vi "Set Test information.vi"(4 "Test Information In":T1={"Scan barcode"=FALSE, "Length"=0, "Test Station Code"="", "Environment"="", "Inspector"="", "Customer Name"="", "Order Number"="", "Fail Rate Max"=0.0, "Repeat"=10}) -> (1 "Test Information":T1={"Scan barcode"=FALSE, "Length"=0, "Test Station Code"="", "Environment"="", "Inspector"="", "Customer Name"="", "Order Number"="", "Fail Rate Max"=0.0, "Repeat"=10})   [LabVIEW 2018]
uses:
  <vilib>/Utility/config.llb/Write Key (String).vi
  <vilib>/Utility/config.llb/NI_LVConfig.lvlib
panel:
  in  "保存路径":bool
  in  "customname 2":string caption="夹具编号"
  out "元素 4":bool
  out "元素 3":bool
  out "元素 2":bool
  out "元素":bool
  in  "XML":bool
  in  "TXT":bool
  in  "CSV":bool
  in  "MES":bool
  out "数组":string[](array[string])
  out "添加的路径":path
  out "添加的数组":string[](array[string])
  out "布尔":bool
  in  "Bar":bool
  out "exit":bool
  in  "重测":i32=10 caption="Max"
  in  "count":string caption="检 验 员"
  in  "SCAN":bool
  in  "长度":u8=8 min=1
  in  "不超过":dbl=10.0 caption="Max" format="%#.2f"
  in  "Cancel":bool
  in  "OK":bool
  in  "envirment":string caption="测试环境"
  in  "order":string caption="工    令"
  in  "customname":string caption="测试计数"
  in  "是否扫条形码":bool
  # "SetTestInformaton"
  # "不良率报警设置"
  # "信息设置"
  # "字符"
  # "%"
  # "提示：勾选了扫描条码，但其长度设置为0表示不校验输入条码。"
  # "数据保存位置"
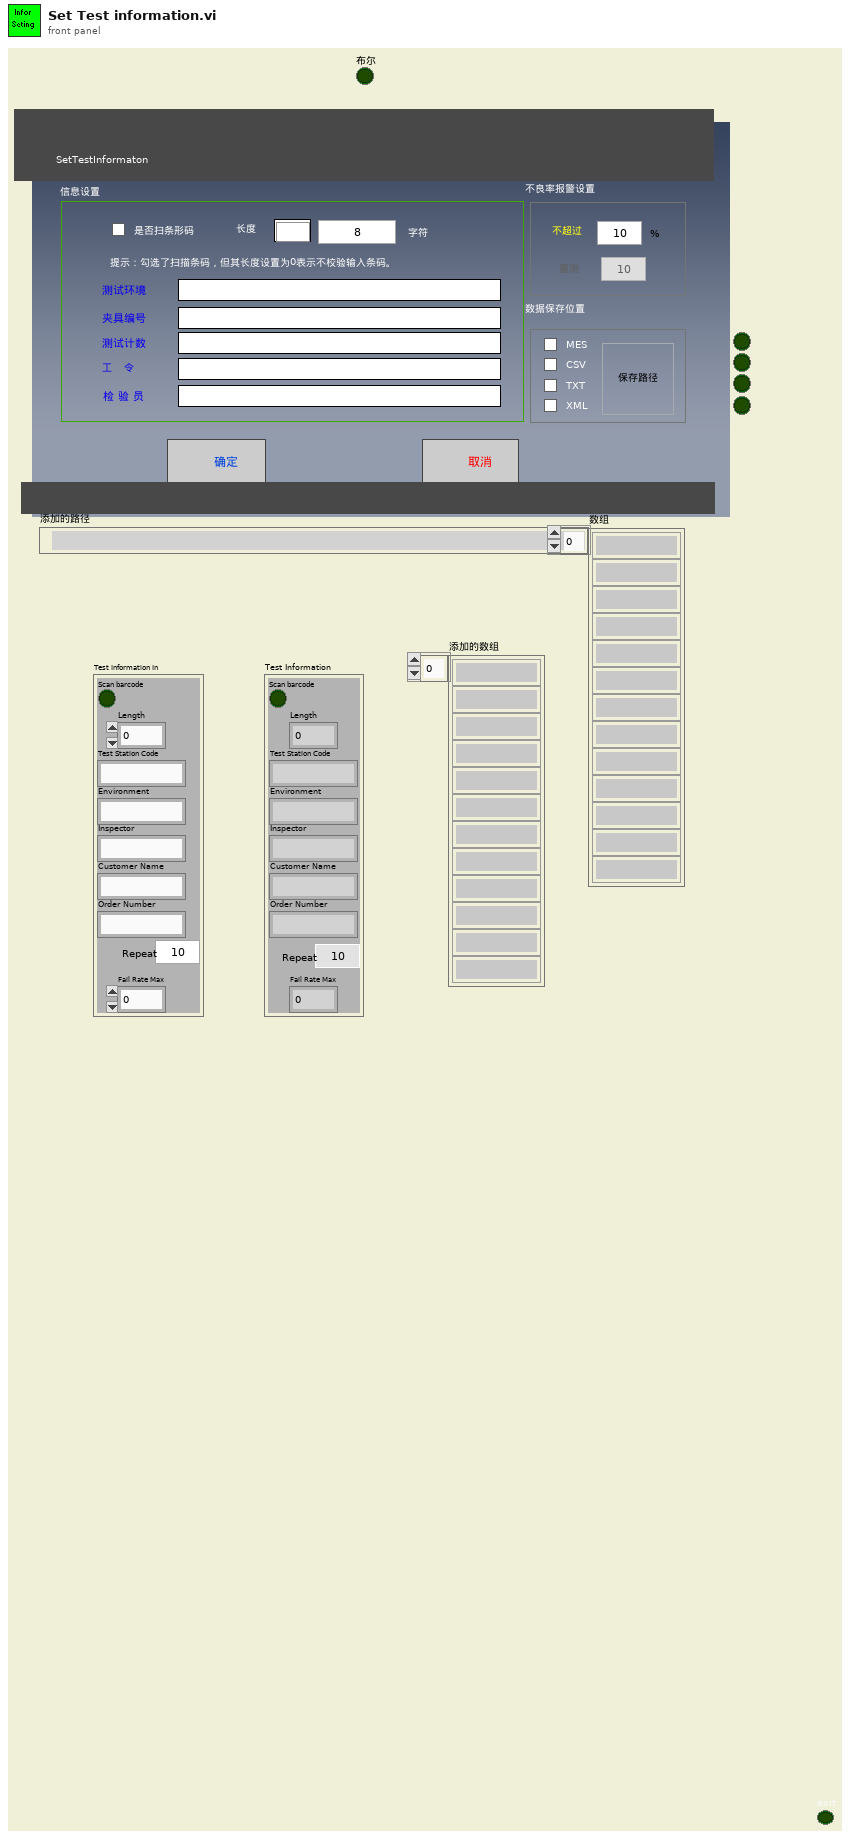
[diagram p1: front panel]
types:
  T1 = cluster{"Scan barcode":bool, "Length":u8, "Test Station Code":string, "Environment":string, "Inspector":string, "Customer Name":string, "Order Number":string, "Fail Rate Max":dbl, "Repeat":i32}
  T2 = typedef "NI_LVConfig.lvlib/Config Data RefNum.ctl" = refnum<k1>
  T3 = cluster{"Scan barcode":bool, "Length":u8, "Test Station Code":string, "Environment":string, "Inspector":string, "Customer Name":string, "Order Number":string, "Fail Rate Max":dbl, "repeat":i32}
  T4 = typedef "Window Refnum.ctl" = refnum<k1>
  T5 = typedef "Window Rectangle.ctl" = cluster{"left":i16, "top":i16, "right":i16, "bottom":i16}
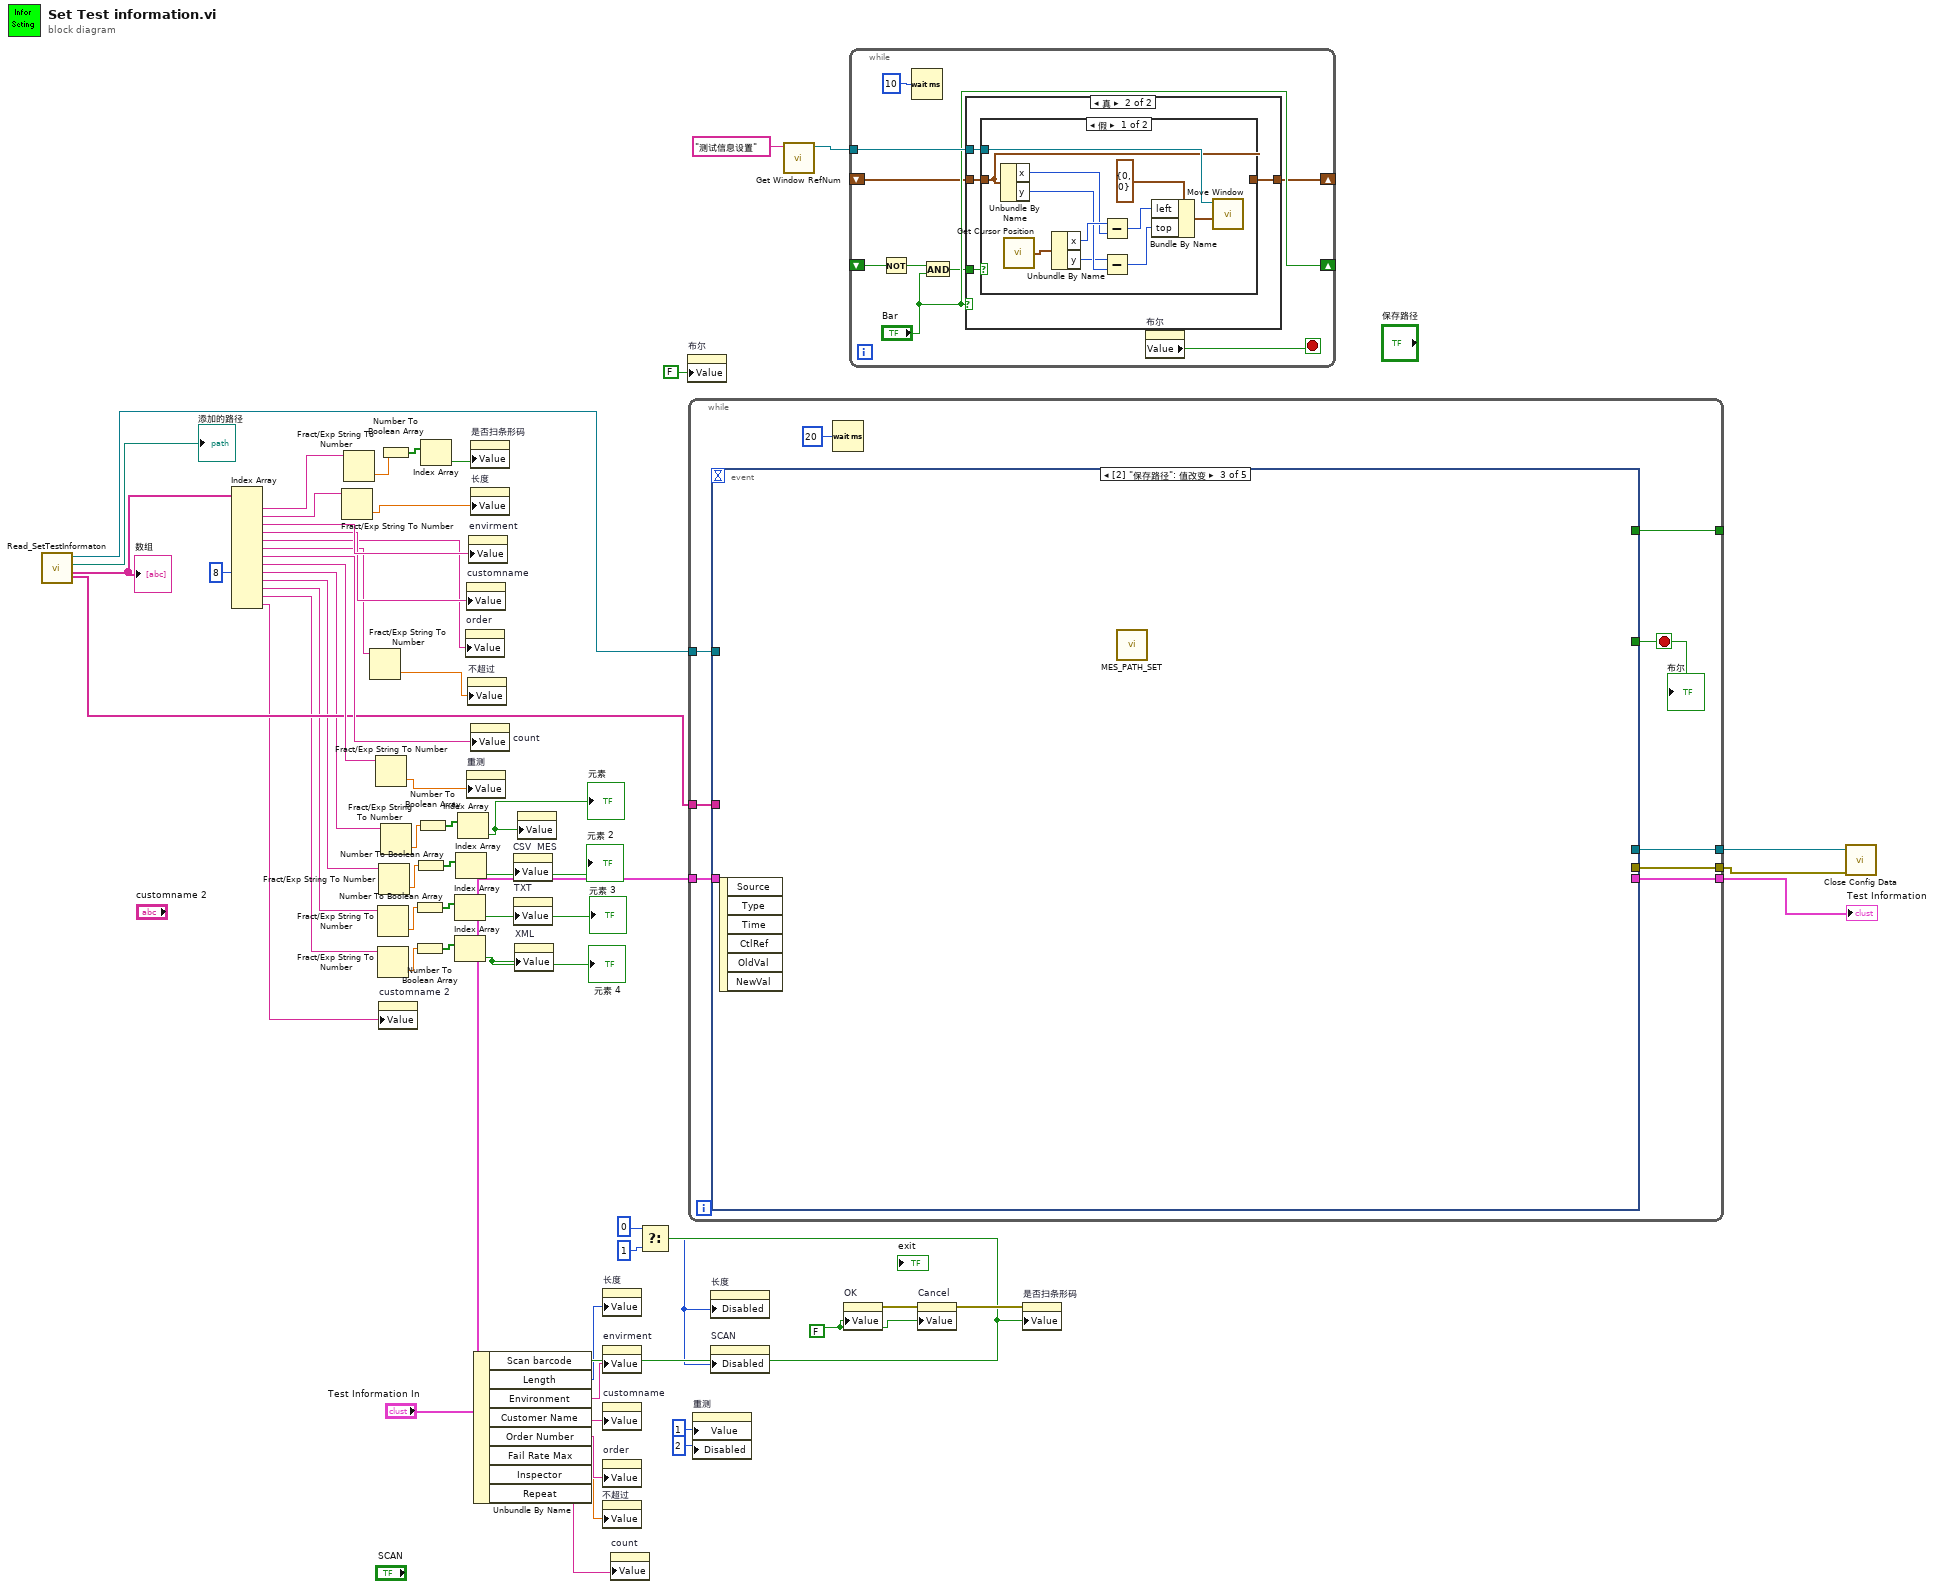
[diagram p0: block diagram]
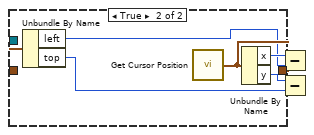
[diagram p3: hidden frame]
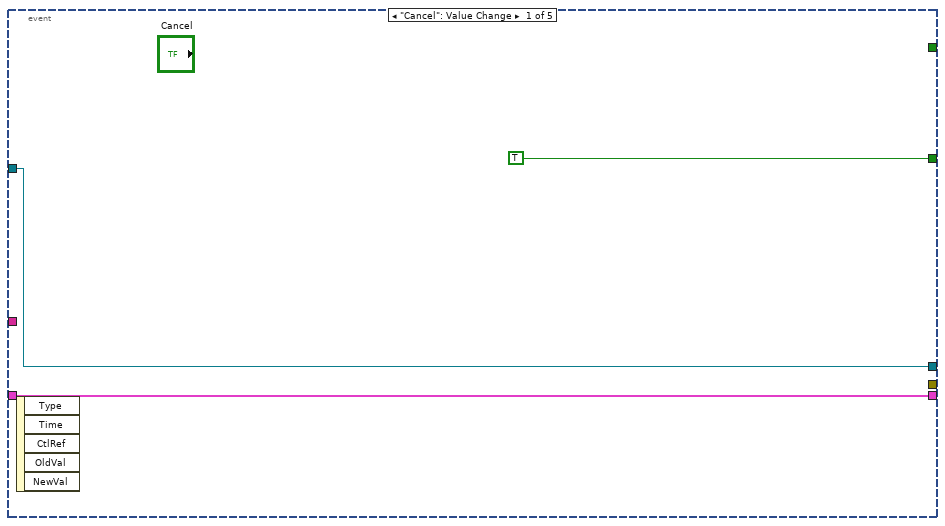
[diagram p4: hidden frame]
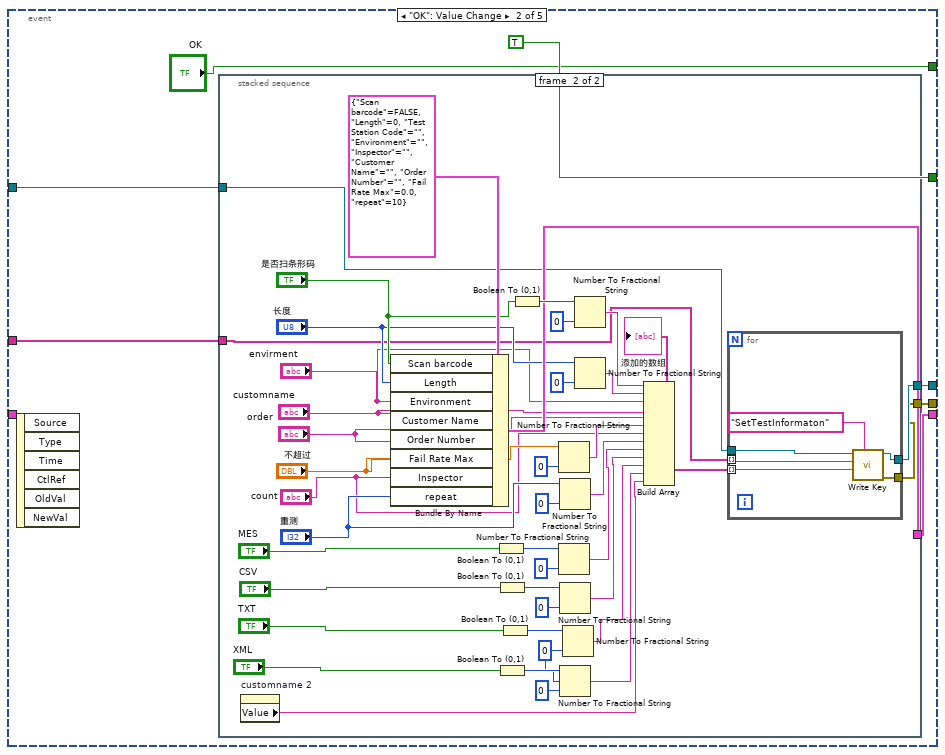
[diagram p5: hidden frame]
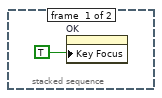
[diagram p6: hidden frame]
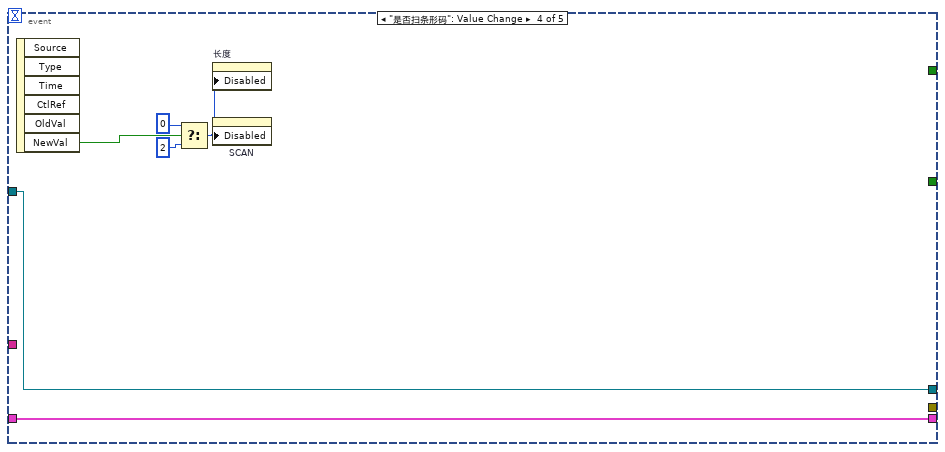
[diagram p7: hidden frame]
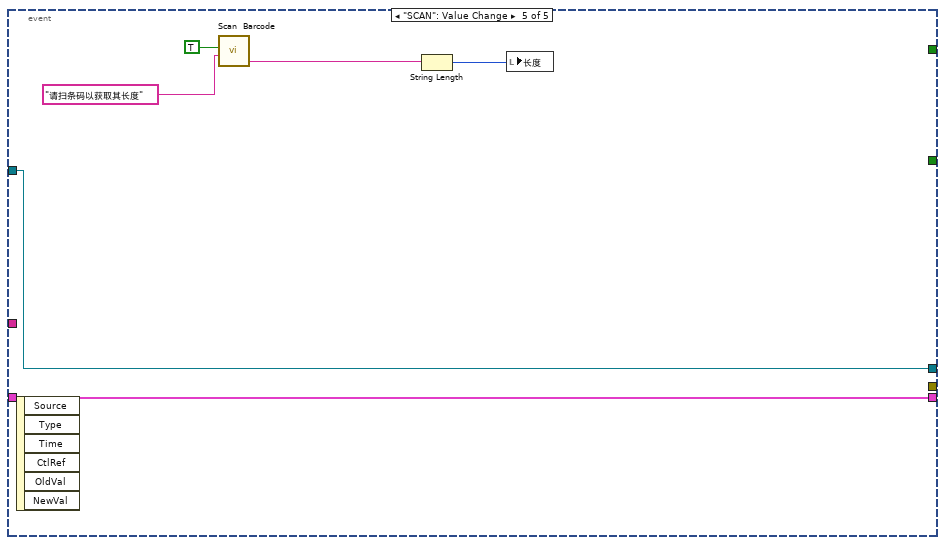
[diagram p8: hidden frame]
diagram:
  w57 = FALSE
  n1 = call "Read_SetTestInformaton.vi"() -> ("数组 2"=w36:string[], "appended path"=→"添加的路径":path, "引用句柄输出"=w37:T2, "数组"=w21:string[])  [unwired: 7 in, 1 out]
  "数组" <- w36
  n2 = Index Array(array=w36, index #9=8 ("索引")) -> (element #1=w35:string, element #2=w31:string, element #3=w29:string, element #4=w28:string, element #5=w27:string, element #6=w25:string, element #7=w24:string, element #8=w22:string, element #9=w14:string, element #10=w13:string, element #11=w12:string, element #12=w11:string, element #13=w1:string)  [unwired: 12 in]
  n3 = Fract/Exp String To Number(string=w31) -> (number=w30:dbl)  [unwired: 3 in, 1 out]
  n4 = Fract/Exp String To Number(string=w35) -> (number=w34:dbl)  [unwired: 3 in, 1 out]
  n5 = Fract/Exp String To Number(string=w25) -> (number=w26:dbl)  [unwired: 3 in, 1 out]
  n6 = Fract/Exp String To Number(string=w22) -> (number=w23:dbl)  [unwired: 3 in, 1 out]
  n7 = Fract/Exp String To Number(string=w12) -> (number=w3:dbl)  [unwired: 3 in, 1 out]
  n8 = Fract/Exp String To Number(string=w11) -> (number=w2:dbl)  [unwired: 3 in, 1 out]
  n9 = Fract/Exp String To Number(string=w13) -> (number=w4:dbl)  [unwired: 3 in, 1 out]
  n10 = property on="customname 2" class="Str"("Value"=w1) -> ()  [unwired: 2 in, 2 out]
  n11 = Number To Boolean Array(number=w34) -> (Boolean array=w33:bool[])
  n12 = Fract/Exp String To Number(string=w14) -> (number=w5:dbl)  [unwired: 3 in, 1 out]
  n13 = Number To Boolean Array(number=w3) -> (Boolean array=w16:bool[])
  n14 = Number To Boolean Array(number=w2) -> (Boolean array=w15:bool[])
  n15 = Number To Boolean Array(number=w4) -> (Boolean array=w17:bool[])
  n16 = Number To Boolean Array(number=w5) -> (Boolean array=w18:bool[])
  n17 = Index Array(array=w33) -> (element=w32:bool)  [unwired: 1 in]
  n18 = Index Array(array=w16) -> (element=w9:bool)  [unwired: 1 in]
  "元素 3" <- w9
  n19 = Index Array(array=w15) -> (element=w10:bool)  [unwired: 1 in]
  "元素 4" <- w10
  n20 = Index Array(array=w17) -> (element=w8:bool)  [unwired: 1 in]
  "元素 2" <- w8
  n21 = Index Array(array=w18) -> (element=w7:bool)  [unwired: 1 in]
  "元素" <- w7
  n22 = property on="order" class="Str"("Value"=w27) -> ()  [unwired: 2 in, 2 out]
  n23 = property on="customname" class="Str"("Value"=w28) -> ()  [unwired: 2 in, 2 out]
  n24 = property on="重测" class="DigNum (严格)"("Value"=w23) -> ()  [unwired: 2 in, 2 out]
  n25 = property on="不超过" class="DigNum (严格)"("Value"=w26) -> ()  [unwired: 2 in, 2 out]
  n26 = property on="envirment" class="Str"("Value"=w29) -> ()  [unwired: 2 in, 2 out]
  n27 = property on="是否扫条形码" class="Bool (严格)"("Value"=w32) -> ()  [unwired: 2 in, 2 out]
  n28 = property on="长度" class="DigNum (严格)"("Value"=w30) -> ()  [unwired: 2 in, 2 out]
  n29 = property on="count" class="Str"("Value"=w24) -> ()  [unwired: 2 in, 2 out]
  n30 = Unbundle By Name("Test Information In") -> ("Scan barcode"=w51:bool, "Length"=w47:u8, "Environment"=w56:string, "Customer Name"=w55:string, "Order Number"=w54:string, "Fail Rate Max"=w46:dbl, "Inspector"=w45:string)  [unwired: 1 out]
  n31 = property on="CSV" class="Bool (严格)"("Value"=w8) -> ()  [unwired: 2 in, 2 out]
  n32 = property on="TXT" class="Bool (严格)"("Value"=w9) -> ()  [unwired: 2 in, 2 out]
  n33 = property on="XML" class="Bool (严格)"("Value"=w10) -> ()  [unwired: 2 in, 2 out]
  n34 = property on="MES" class="Bool (严格)"("Value"=w7) -> ()  [unwired: 2 in, 2 out]
  n35 = property on="长度" class="DigNum (严格)"("Value"=w47) -> ()  [unwired: 2 in, 2 out]
  n36 = property on="envirment" class="Str"("Value"=w56) -> ()  [unwired: 2 in, 2 out]
  n37 = property on="customname" class="Str"("Value"=w55) -> ()  [unwired: 2 in, 2 out]
  n38 = property on="order" class="Str"("Value"=w54) -> ()  [unwired: 2 in, 2 out]
  n39 = property on="不超过" class="DigNum (严格)"("Value"=w46) -> ()  [unwired: 2 in, 2 out]
  n40 = property on="count" class="Str"("Value"=w45) -> ()  [unwired: 2 in, 2 out]
  n41 = Select(t=u8 0 ("禁用"), s=w51, f=u8 1 ("禁用")) -> (s? t:f=w48:u8)
  n42 = property on="布尔" class="Bool (严格)"("Value"=FALSE ("布尔")) -> ()  [unwired: 2 in, 2 out]
  n43 = while {
    tunnel: [w62] -> w39
    tunnel: "Test Information In" -> [w65]
    tunnel: [w64] -> _
    tunnel: w37 -> [w59]
    tunnel: w21 -> [w63]
    tunnel: [w61] -> w20
    tunnel: [w60] -> w19
    stop <- w66 stop-if-true
    n44 = event shown="[2] \"保存路径\": 值改变" {
      selector: _ -> [_ _ _ _ _]
      dyn-events: _ -> [_ _ _ _ _]
      timeout: _ -> [_ _ _ _ _]
      tunnel: [TRUE TRUE _ _ _] -> w66
      tunnel: [w69 w71 _ w127 w135] -> w62
      tunnel: w65 -> [w69 _ _ w127 w135]
      tunnel: [_ "OK" _ _ _] -> w64
      tunnel: w63 -> [_ w75 _ _ _]
      tunnel: [w68 w74 _ w126 w132] -> w61
      tunnel: [_ w73 _ _ _] -> w60
      tunnel: w59 -> [w68 w72 _ w126 w132]
      event "Cancel": Value Change {
        n45 = event-data() -> ()  [unwired: 6 out]
      }
      event "OK": Value Change {
        n46 = event-data() -> ()  [unwired: 7 out]
        n47 = stacked-sequence {
          tunnel: w75 -> [_ w100]
          tunnel: [_ w109] -> w74
          tunnel: [_ w108] -> w73
          tunnel: w72 -> [_ w101]
          tunnel: [_ w107] -> w71
          frame #0 {
            n48 = property on="OK" class="Bool (严格)"("Key Focus"=TRUE) -> ()  [unwired: 2 in, 2 out]
          }
          frame #1 {
            w88 = i16 0 ("精度(6)")
            n49 = property on="customname 2" class="Str"() -> ("Value"=w79:string)  [unwired: 2 in, 2 out]
            n50 = Bundle By Name(cluster=T3 {"Scan barcode"=FALSE, "Length"=0, "Test Station Code"="", "Environment"="", "Inspector"="", "Customer Name"="", "Order Number"="", "Fail Rate Max"=0.0, "repeat"=10} ("Test Information In 2"), "Scan barcode"="是否扫条形码", "Length"="长度", "Environment"="envirment", "Customer Name"="customname", "Order Number"="order", "Fail Rate Max"="不超过", "Inspector"="count", "repeat"="重测") -> (w107:T3)
            n51 = Boolean To (0,1)(Boolean="MES") -> (0, 1=w94:i16)
            n52 = Boolean To (0,1)(Boolean="CSV") -> (0, 1=w93:i16)
            n53 = Boolean To (0,1)(Boolean="XML") -> (0, 1=w90:i16)
            n54 = Boolean To (0,1)(Boolean="TXT") -> (0, 1=w91:i16)
            n55 = Boolean To (0,1)(Boolean="是否扫条形码") -> (0, 1=w114:i16)
            n56 = Number To Fractional String(number="不超过", precision (6)=i16 0 ("精度(6)")) -> (F-format string=w97:string)  [unwired: 2 in]
            n57 = Number To Fractional String(number=w94, precision (6)=i16 0 ("精度(6)")) -> (F-format string=w87:string)  [unwired: 2 in]
            n58 = Number To Fractional String(number="重测", precision (6)=i16 0 ("精度(6)")) -> (F-format string=w117:string)  [unwired: 2 in]
            n59 = Number To Fractional String(number=w93, precision (6)=i16 0 ("精度(6)")) -> (F-format string=w86:string)  [unwired: 2 in]
            n60 = Number To Fractional String(number=w90, width (-)=w88, precision (6)=i16 0 ("精度(6)")) -> (F-format string=w84:string)  [unwired: 1 in]
            n61 = Number To Fractional String(number=w91, precision (6)=w88) -> (F-format string=w85:string)  [unwired: 2 in]
            n62 = Number To Fractional String(number=w114, precision (6)=i16 0 ("精度(6)")) -> (F-format string=w115:string)  [unwired: 2 in]
            n63 = Number To Fractional String(number="长度", precision (6)=i16 0 ("精度(6)")) -> (F-format string=w116:string)  [unwired: 2 in]
            n64 = Build Array(w115, w116, "envirment", "customname", "order", w97, "count", w117, w87, w86, w85, w84, w79) -> (w118:string[])
            "添加的数组" <- w118
            n65 = for {
              tunnel: w100 -> [w124] mode=indexing
              tunnel: w118 -> [w125] mode=indexing
              tunnel: [w122] -> w109
              tunnel: [w121] -> w108
              tunnel: w101 -> [w120]
              n66 = call-poly <vilib>:"Write Key.vi"("section"="SetTestInformaton", "value"=w125, "key"=w124, "refnum"=w120) -> ("error out"=w121:errorcluster, "refnum out"=w122:T2)  [unwired: 5 in, 1 out]
            }
          }
        }
      }
      event "保存路径": Value Change {
        n67 = event-data() -> ()  [unwired: 7 out]
        n68 = call "MES_PATH_SET.vi"() -> ()  [unwired: 12 in]
      }
      event "是否扫条形码": Value Change {
        n69 = event-data() -> ("NewVal"=w131:bool)  [unwired: 6 out]
        n70 = Select(t=u8 0 ("禁用"), s=w131, f=u8 2 ("禁用")) -> (s? t:f=w128:u8)
        n71 = property on="长度" class="DigNum (严格)"("Disabled"=w128) -> ()  [unwired: 2 in, 2 out]
        n72 = property on="SCAN" class="Bool"("Disabled"=w128) -> ()  [unwired: 2 in, 2 out]
      }
      event "SCAN": Value Change {
        n73 = event-data() -> ()  [unwired: 7 out]
        n74 = call "Scan  Barcode.vi"("前面板窗口:标题"="请扫条码以获取其长度", "no check?"=TRUE ("检查否")) -> ("SN"=w137:string)  [unwired: 2 in, 2 out]
        n75 = String Length(string=w137) -> (length=w136:i32)
        n76 = local write "长度"(w136) -> ()
      }
    }
    "布尔" <- w66
    n77 = Wait (ms)(milliseconds to wait=u32 20) -> ()  [unwired: 1 out]
  }
  "Test Information" <- w39
  n78 = property on="重测" class="DigNum (严格)"("Value"=1 ("重测"), "Disabled"=u8 2 ("禁用")) -> ()  [unwired: 2 in, 2 out]
  n79 = property on="长度" class="DigNum (严格)"("Disabled"=w48) -> ()  [unwired: 2 in, 2 out]
  n80 = property on="SCAN" class="Bool"("Disabled"=w48) -> ()  [unwired: 2 in, 2 out]
  n81 = call "Get Window RefNum.vi"("window name (\"\")"="测试信息设置" ("window name (\"\")")) -> ("window refnum (NaWR)"=w41:T4)  [unwired: 1 in, 7 out]
  n82 = property on="OK" class="Bool (严格)"("Value"=w57) -> (error out=w58:errorcluster)  [unwired: 2 in, 1 out]
  n83 = while {
    shift-left: _ -> [w140]
    shift-right: [w141] -> _
    shift-left: _ -> [w144]
    shift-right: ["Bar"] -> _
    tunnel: w41 -> [w145]
    stop <- w138 stop-if-true
    n84 = Not(x=w144) -> (.not. x?=w143:bool)
    n85 = Wait (ms)(milliseconds to wait=u32 10) -> ()  [unwired: 1 out]
    n86 = And(x=w143, y="Bar") -> (x .and. y?=w139:bool)
    n87 = case shown="真" "Bar" {
      tunnel: w145 -> [_ w151]
      tunnel: [w147 w150] -> w141
      tunnel: w140 -> [w147 w148]
      tunnel: w139 -> [_ w149]
      frame False {
      }
      frame True {
        n88 = case shown="假" w149 {
          tunnel: w151 -> [w157 w173]
          tunnel: [w152 w163] -> w150
          tunnel: w148 -> [w152 _]
          frame False {
            n89 = Unbundle By Name(w152) -> ("x"=w160:i16, "y"=w159:i16)
            n90 = call "Get Cursor Position.vi"() -> ("cursor position"=w162:cluster{"x":i16, "y":i16})
            n91 = Unbundle By Name(w162) -> ("x"=w161:i16, "y"=w158:i16)
            n92 = Subtract(x=w161, y=w160) -> (x-y=w154:i16)
            n93 = Subtract(x=w158, y=w159) -> (x-y=w155:i16)
            n94 = Bundle By Name(cluster=cluster{"left":i16, "top":i16} {"left"=0, "top"=0} ("new position (0,0)"), "left"=w154, "top"=w155) -> (w153:cluster{"left":i16, "top":i16})
            n95 = call "Move Window.vi"("new position (0,0)"=w153, "window refnum (NaWR)"=w157) -> ()  [unwired: 2 in, 4 out]
          }
          frame True {
            n96 = call "Get Window Rectangle.vi"("window refnum (NaWR)"=w173) -> ("window rect"=w172:T5)  [unwired: 1 in, 5 out]
            n97 = call "Extract Window Origin.vi"("window rect"=w172) -> ("window origin"=w171:cluster{"left":i16, "top":i16})  [unwired: 1 out]
            n98 = Unbundle By Name(w171) -> ("left"=w168:i16, "top"=w167:i16)
            n99 = call "Get Cursor Position.vi"() -> ("cursor position"=w170:cluster{"x":i16, "y":i16})
            n100 = Unbundle By Name(w170) -> ("x"=w169:i16, "y"=w166:i16)
            n101 = Subtract(x=w169, y=w168) -> (x-y=w164:i16)
            n102 = Subtract(x=w166, y=w167) -> (x-y=w165:i16)
            n103 = Bundle By Name(cluster=w170, "x"=w164, "y"=w165) -> (w163:cluster{"x":i16, "y":i16})
          }
        }
      }
    }
    n104 = property on="布尔" class="Bool (严格)"() -> ("Value"=w138:bool)  [unwired: 2 in, 2 out]
  }
  n105 = property on="Cancel" class="Bool (严格)"(error in=w58, "Value"=w57) -> (error out=w53:errorcluster)  [unwired: 1 in, 1 out]
  n106 = property on="是否扫条形码" class="Bool (严格)"(error in=w53, "Value"=w51) -> ()  [unwired: 1 in, 2 out]
  n107 = call <vilib>:"Close Config Data.vi"("error in (no error)"=w19, "refnum"=w20) -> ()  [unwired: 8 in, 2 out]
